vi "_script_remove_all_csm_bookmarks.vi"(11 "vi path":path=path "D:/github/JKI-State-Machine-Plus/src/user.lib/_NEVSTOP/JKI State Machine++/JKISM++ No-Event Structure Template.vi") -> ()   [LabVIEW 2017]
uses:
  _csmHelper/API/Destroy.vi
  _csmHelper/API/Stop Undo.vi
  _csmHelper/Properties/Read Block Diagram Ref.vi
  _csmHelper/API/Start Undo.vi
  _csmHelper/API/Open Block Diagram.vi
  _csmHelper/API/Create From VI Reference.vi
  _csmHelper/CSM-Helper.lvclass
  _csmHelper/Properties/Read VI Ref.vi
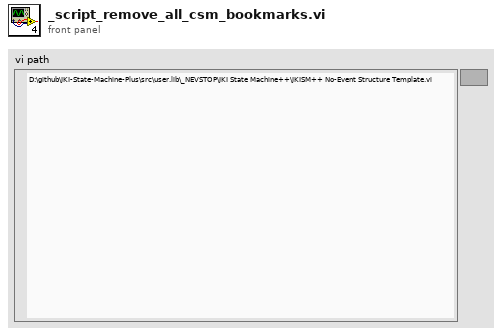
[diagram p1: front panel]
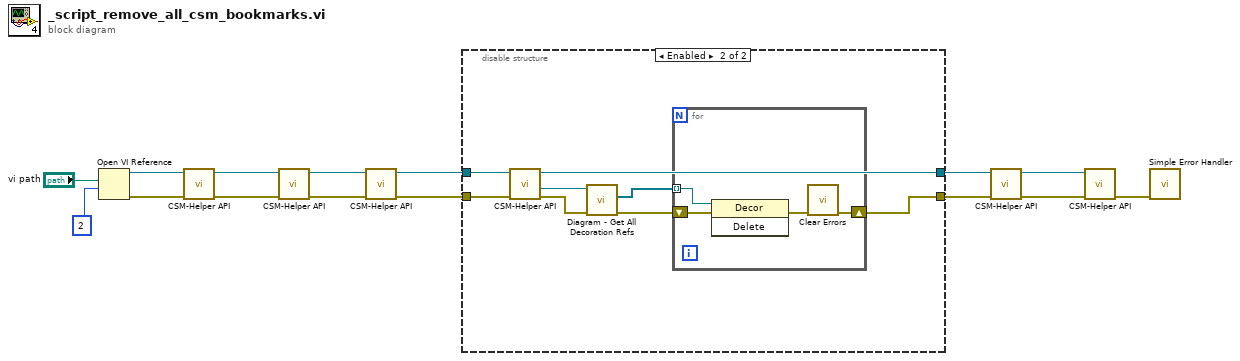
[diagram p0: block diagram]
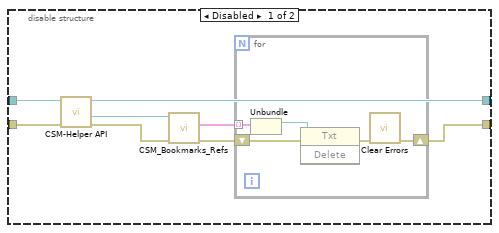
[diagram p2: hidden frame]
diagram:
  n1 = Open VI Reference(vi path="vi path", options=2) -> (vi reference=w13:refnum<vi>, error out=w12:errorcluster)  [unwired: 4 in]
  n2 = call-poly "CSM-Helper API.vi"("error in (no error)"=w12, "VI"=w13) -> ("error out"=w11:errorcluster, "CSM-Helper.lvclass"=w10:refnum<class "CSM-Helper.lvclass">)  [unwired: 8 in]
  n3 = call-poly "CSM-Helper API.vi"("error in (no error)"=w11, "CSM-Helper in"=w10) -> ("error out"=w9:errorcluster, "CSM-Helper out"=w8:refnum<class "CSM-Helper.lvclass">)  [unwired: 8 in]
  n4 = call-poly "CSM-Helper API.vi"("error in (no error)"=w9, "CSM-Helper in"=w8) -> ("error out"=w7:errorcluster, "CSM-Helper out"=w6:refnum<class "CSM-Helper.lvclass">)  [unwired: 8 in]
  n5 = disable-structure shown="Enabled" {
    disable-tunnel: w7 -> [w19 w36]
    disable-tunnel: w6 -> [w18 w35]
    disable-tunnel: [w17 w29] -> w5
    disable-tunnel: [w16 w30] -> w4
    frame Disabled {
      n6 = call-poly "CSM-Helper API.vi"("error in (no error)"=w19, "CSM-Helper in"=w18) -> ("error out"=w20:errorcluster, "VI"=w21:refnum<vi>, "CSM-Helper out"=w16:refnum<class "CSM-Helper.lvclass">)  [unwired: 7 in]
      n7 = call "CSM_Bookmarks_Refs.vi"("error in (no error)"=w20, "VIRef"=w21) -> ("error out"=w22:errorcluster, "Array"=w23:cluster{refnum<vi>, "Text":string}[])  [unwired: 7 in, 1 out]
      n8 = for {
        tunnel: w23 -> [w28] mode=indexing
        shift-right: [w24] -> w17
        shift-left: w22 -> [w26]
        n9 = Unbundle(w28) -> (w27:refnum<vi>)  [unwired: 1 out]
        n10 = invoke class="Txt" method="Delete"(reference=w27, error in=w26) -> (error out=w25:errorcluster)  [unwired: 1 in, 2 out]
        n11 = call <vilib>:"Clear Errors.vi"("error in (no error)"=w25) -> ("error out"=w24:errorcluster)  [unwired: 5 in, 1 out]
      }
    }
    frame Enabled {
      n12 = call-poly "CSM-Helper API.vi"("error in (no error)"=w36, "CSM-Helper in"=w35) -> ("error out"=w34:errorcluster, "Diagram"=w33:refnum<vi>, "CSM-Helper out"=w30:refnum<class "CSM-Helper.lvclass">)  [unwired: 7 in]
      n13 = call "Diagram - Get All Decoration Refs.vi"("error in (no error)"=w34, "TopLevelDiagram in"=w33) -> ("error out"=w32:errorcluster, "TextRefs"=w31:refnum<vi>[])  [unwired: 7 in, 1 out]
      n14 = for {
        shift-right: [w38] -> w29
        shift-left: w32 -> [w40]
        tunnel: w31 -> [w37] mode=indexing
        n15 = invoke class="Decor" method="Delete"(reference=w37, error in=w40) -> (error out=w39:errorcluster)  [unwired: 1 in, 2 out]
        n16 = call <vilib>:"Clear Errors.vi"("error in (no error)"=w39) -> ("error out"=w38:errorcluster)  [unwired: 5 in, 1 out]
      }
    }
  }
  n17 = call-poly "CSM-Helper API.vi"("error in (no error)"=w5, "CSM-Helper in"=w4) -> ("error out"=w3:errorcluster, "CSM-Helper out"=w2:refnum<class "CSM-Helper.lvclass">)  [unwired: 8 in]
  n18 = call-poly "CSM-Helper API.vi"("error in (no error)"=w3, "CSM-Helper in"=w2) -> ("error out"=w1:errorcluster)  [unwired: 8 in, 1 out]
  n19 = call <vilib>:"Simple Error Handler.vi"("error in (no error)"=w1) -> ()  [unwired: 4 in, 5 out]
